vi "Make Vertical-set ROLL.vi"(8 "Roll":dbl, 11 "Matrix":T1 format="%.3f") -> (3 "Vertical Matrix":T1 format="%.3f")   [LabVIEW 2013]
uses:
  <vilib>/Analysis/Matrix/Datatypes/RealMatrix.ctl
  <vilib>/Analysis/Matrix/Numeric/Conversions/Array To Matrix - RA2.vi
  <vilib>/Analysis/Matrix/Numeric/Multiply/Multiply - RM,RM.vi
  <vilib>/Analysis/Matrix/NI_Matrix.lvlib
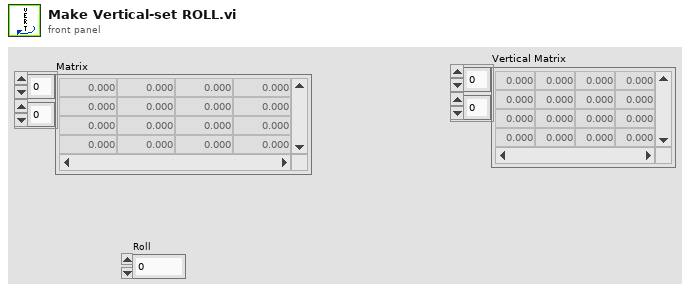
[diagram p1: front panel]
types:
  T1 = typedef "NI_Matrix.lvlib/RealMatrix.ctl" = dbl[][]
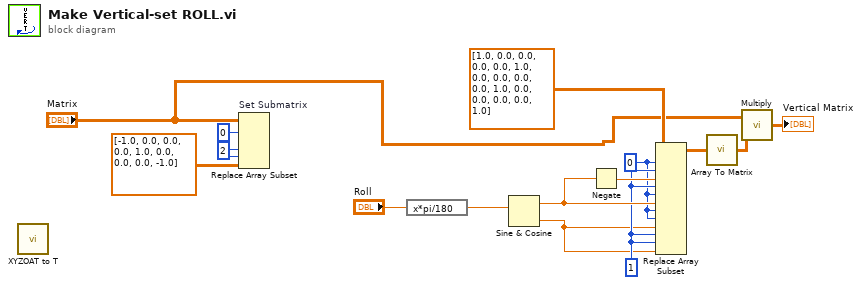
[diagram p0: block diagram]
diagram:
  w14 = 2 ("row N")
  w15 = 0 ("row 1")
  w4 = 1 ("disabled index (col)")
  w3 = 0 ("index (row)")
  n1 = call "XYZOAT to T.vi"() -> ()  [unwired: 11 in, 1 out]
  n2 = Replace Array Subset "Set Submatrix"(array="Matrix", new element=dbl[][] [[-1.0, 0.0, 0.0], [0.0, 1.0, 0.0], [0.0, 0.0, -1.0]], index (dim 0)=w15, index (dim 1)=w14, index (dim 2)=w15, index (dim 3)=w14) -> ()  [unwired: 1 out]
  n3 = expression code="x*pi/180"("Roll") -> (w8:dbl)
  n4 = Sine & Cosine(0:w8) -> (1:w5:dbl, 2:w2:dbl)
  n5 = Negate(x=w5) -> (-x=w6:dbl)
  n6 = Replace Array Subset(array=dbl[][] [[1.0, 0.0, 0.0, 0.0], [0.0, 1.0, 0.0, 0.0], [0.0, 0.0, 1.0, 0.0], [0.0, 0.0, 0.0, 1.0]], new element #1=w6, index (row) #1=w3, index (col) #1=w4, new element #2=w5, index (row) #2=w4, index (col) #2=w3, new element #3=w2, index (row) #3=w3, index (col) #3=w3, new element #4=w2, index (row) #4=w4, index (col) #4=w4) -> (w11:dbl[][])
  n7 = call-poly <vilib>:"Array To Matrix.vi"("Real 2D Array"=w11) -> ("Real Matrix"=w10:T1)
  n8 = call-poly <vilib>:"Multiply.vi"("Real Matrix B"=w10, "Real Matrix A"="Matrix") -> ("A * B"=→"Vertical Matrix":T1)
